vi "Update Common Items.vi"(8 "error in (no error)":errorcluster, 10 "NewVal":T1, 11 "ColumnPanel in":refnum<class "ColumnPanel.lvclass">) -> (0 "error out":errorcluster, 3 "ColumnPanel out":refnum<class "ColumnPanel.lvclass">)   [LabVIEW 2020, in "Conditum-Tools.lvlib" / "ColumnPanel.lvclass"]
uses:
  ColumnPanel.lvclass
  Common Items.ctl
  Accessors.ctl
  Accessor Scope.ctl
  Conditum-Clone/Attributes.ctl
  Conditum-Clone/Columns/Type/Definition.ctl
  Conditum-Clone/Conditu2.lvlib
  Conditum-Clone/Columns/Type/Type.lvclass
  Conditum-Tools.lvlib
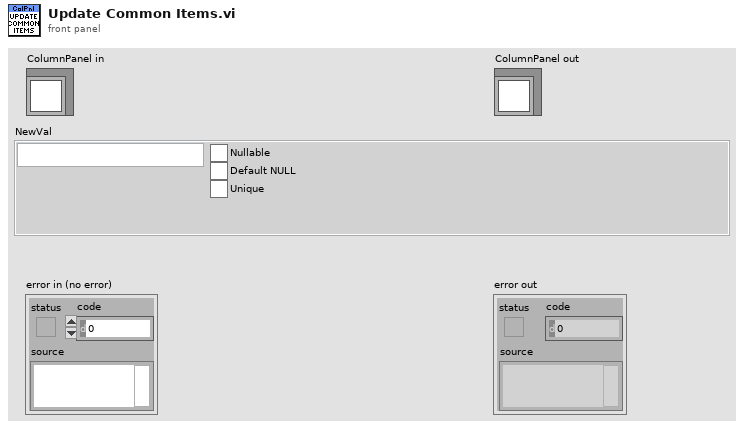
[diagram p1: front panel]
types:
  T1 = typedef "Conditum-Tools.lvlib/ColumnPanel.lvclass/Common Items.ctl" = cluster{"Name":string, "Nullable":bool, "Default NULL":bool, "Unique":bool, "Accessors":T2}
  T2 = typedef "Conditum-Tools.lvlib/Accessors.ctl" = cluster{"Get":T3, "Set":T3}
  T3 = typedef "Conditum-Tools.lvlib/Accessor Scope.ctl" = enum16{"None", "Public", "Protected", "Private"}
  T4 = typedef "Conditu2.lvlib/Columns.lvlib/Type.lvclass/Definition.ctl" = cluster{"Name":string, "Nullable":bool, "Default NULL":bool}
  T5 = typedef "Conditu2.lvlib/Attributes.ctl" = cluster{"Primary Key":bool, "Unique":bool, "Foreign Key":bool, "Auto Increment":bool}
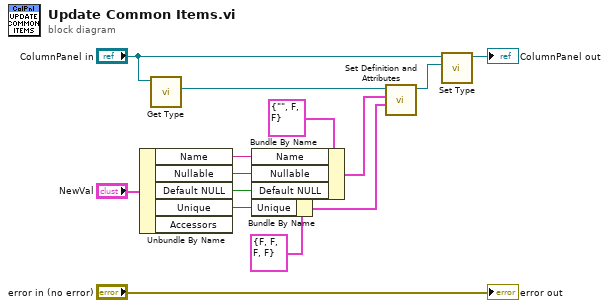
[diagram p0: block diagram]
diagram:
  n1 = Unbundle By Name("NewVal") -> ("Name"=w6:string, "Nullable"=w5:bool, "Default NULL"=w4:bool, "Unique"=w10:bool)  [unwired: 1 out]
  n2 = call-dynamic "Get Type.vi"("ColumnPanel in"="ColumnPanel in") -> ("Type"=w9:refnum<class "Type.lvclass">)  [unwired: 10 in]
  n3 = Bundle By Name(cluster=T4 {"Name"="", "Nullable"=FALSE, "Default NULL"=FALSE} ("Definition"), "Name"=w6, "Nullable"=w5, "Default NULL"=w4) -> (w7:T4)
  n4 = Bundle By Name(cluster=T5 {"Primary Key"=FALSE, "Unique"=FALSE, "Foreign Key"=FALSE, "Auto Increment"=FALSE} ("Attributes"), "Unique"=w10) -> (w3:T5)
  n5 = call "Set Definition and Attributes.vi"("Attributes"=w3, "Definition"=w7, "Type in"=w9) -> ("Type out"=w2:refnum<class "Type.lvclass">)  [unwired: 8 in]
  n6 = call-dynamic "Set Type.vi"("Type"=w2, "ColumnPanel in"="ColumnPanel in") -> ("ColumnPanel out"=→"ColumnPanel out":refnum<class "ColumnPanel.lvclass">)  [unwired: 9 in]
  "error out" <- "error in (no error)"
